vi "Override Error.vi"(10 "Error":errorcluster, 11 "Dev Actor in":refnum<class "Dev Actor.lvclass">) -> (3 "Dev Actor out":refnum<class "Dev Actor.lvclass">)   [LabVIEW 2021, in "Dev Actor.lvlib" / "Dev Actor.lvclass"]
uses:
  Dev Actor.lvclass
  Dev Actor.lvclass/Dev Actor.ctl
  Queue Actor/Queue Actor.lvclass
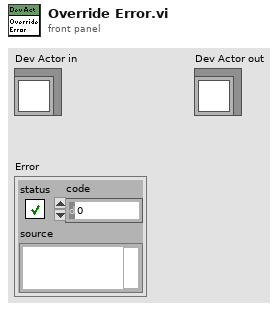
[diagram p1: front panel]
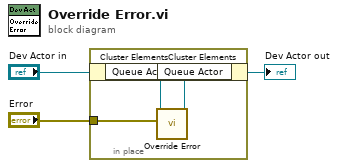
[diagram p0: block diagram]
diagram:
  n1 = in-place {
    in-place-border: "Error" -> [w4]
    n2 = in-place-cluster #1("Dev Actor in") -> ("Queue Actor"=w5:refnum<class "Queue Actor.lvclass">)
    n3 = call-dynamic "Override Error.vi"("Error"=w4, "Override Error in"=w5) -> ("Override Error out"=w6:refnum<class "Queue Actor.lvclass">)  [unwired: 9 in]
    n4 = in-place-cluster #1("Queue Actor"=w6) -> (→"Dev Actor out":refnum<class "Dev Actor.lvclass">)
  }
